vi "NameYScaleTHD (SubVI).vi"(7 "unit labels":T1, 8 "error in (no error)":errorcluster, 9 "XYGraph Refnum 3":refnum<vi>, 10 "XYGraph Refnum in":refnum<vi>, 11 "XYGraph in":refnum<vi>) -> (0 "error out":errorcluster)   [LabVIEW 2018]
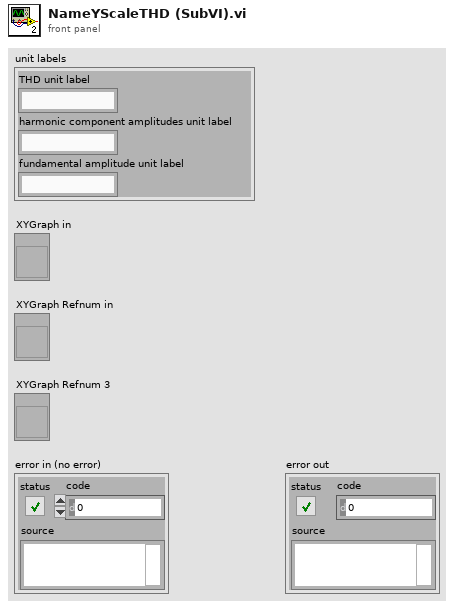
[diagram p1: front panel]
types:
  T1 = cluster{"THD unit label":string, "harmonic component amplitudes unit label":string, "fundamental amplitude unit label":string}
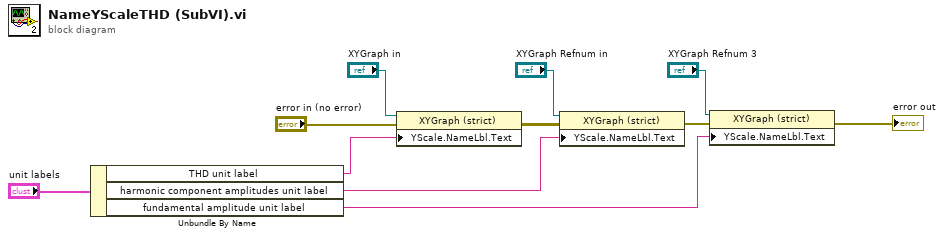
[diagram p0: block diagram]
diagram:
  n1 = Unbundle By Name("unit labels") -> ("THD unit label"=w8:string, "harmonic component amplitudes unit label"=w10:string, "fundamental amplitude unit label"=w11:string)
  n2 = property on="Property Node" class="XYGraph (strict)"(reference="XYGraph in", error in="error in (no error)", "YScale.NameLbl.Text"=w8) -> (error out=w4:errorcluster)  [unwired: 1 out]
  n3 = property on="Property Node" class="XYGraph (strict)"(reference="XYGraph Refnum in", error in=w4, "YScale.NameLbl.Text"=w10) -> (error out=w5:errorcluster)  [unwired: 1 out]
  n4 = property on="Property Node" class="XYGraph (strict)"(reference="XYGraph Refnum 3", error in=w5, "YScale.NameLbl.Text"=w11) -> (error out=→"error out":errorcluster)  [unwired: 1 out]
